vi "Set TCP Info.vi"(8 "error in (no error)":errorcluster, 10 "TCP Messaging Info":T1, 11 "Node in":refnum<class "Node.lvclass">) -> (0 "error out":errorcluster, 3 "Node out":refnum<class "Node.lvclass">)   [LabVIEW 2020, in "VolatusConfig.lvlib" / "Node.lvclass"]
uses:
  Node.lvclass
  Node.lvclass/Node.ctl
  VolatusConfigElement/VolatusConfigElement.lvclass
  lv-cdm/CDM-Config/Config Element/Config Element.lvclass
  lv-cdm/CDM-Config/Value Type.ctl
  lv-cdm/CDM-Config/CDM-Config.lvlib
  C:/dev/lv20CE/relink/lv-volatus/VolatusConfig/VolatusConfigElement/VolatusConfigElement.lvclass
  C:/dev/lv20CE/relink/lv-volatus/VolatusConfig/Node/Node.lvclass
  lv-vecto/Vecto/Node Config/TCP Messaging Info.ctl
  lv-vecto/VectoConfig/VectoConfig.lvlib
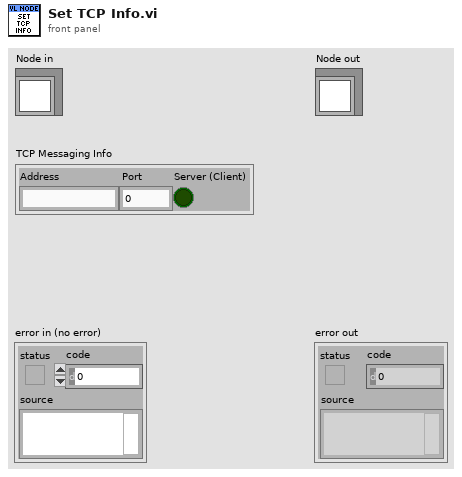
[diagram p1: front panel]
types:
  T1 = typedef "VectoConfig.lvlib/TCP Messaging Info.ctl" = cluster{"Address":string, "Port":u16, "Server (Client)":bool}
  T2 = typedef "CDM-Config.lvlib/Value Type.ctl" = enum16{"String", "Number", "Bool", "Object", "Array"}
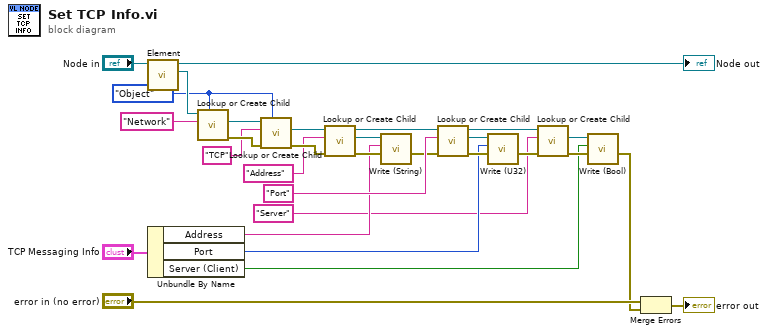
[diagram p0: block diagram]
diagram:
  w23 = Value_Type."Object" ("Value Type (String)")
  n1 = call "Element.vi"("VolatusConfigElement in"="Node in") -> ("Element"=w26:refnum<class "Config Element.lvclass">, "VolatusConfigElement out"=→"Node out":refnum<class "Node.lvclass">)  [unwired: 9 in]
  n2 = Unbundle By Name("TCP Messaging Info") -> ("Address"=w13:string, "Port"=w10:u16, "Server (Client)"=w5:bool)
  n3 = call "Lookup or Create Child.vi"("Value Type (Object)"=w23, "Name"="Network", "Config Element in"=w26) -> ("error out"=w29:errorcluster, "Child"=w24:refnum<class "Config Element.lvclass">)  [unwired: 5 in, 2 out]
  n4 = call "Lookup or Create Child.vi"("Value Type (Object)"=w23, "error in (no error)"=w29, "Name"="TCP", "Config Element in"=w24) -> ("error out"=w20:errorcluster, "Child"=w21:refnum<class "Config Element.lvclass">)  [unwired: 4 in, 2 out]
  n5 = call "Lookup or Create Child.vi"("error in (no error)"=w20, "Name"="Address", "Config Element in"=w21) -> ("error out"=w30:errorcluster, "Child"=w15:refnum<class "Config Element.lvclass">, "Config Element out"=w19:refnum<class "Config Element.lvclass">)  [unwired: 5 in, 1 out]
  n6 = call "Write (String).vi"("error in (no error)"=w30, "String Value"=w13, "Config Element in"=w15) -> ("error out"=w16:errorcluster)  [unwired: 7 in, 1 out]
  n7 = call "Lookup or Create Child.vi"("error in (no error)"=w16, "Name"="Port", "Config Element in"=w19) -> ("error out"=w12:errorcluster, "Child"=w11:refnum<class "Config Element.lvclass">, "Config Element out"=w8:refnum<class "Config Element.lvclass">)  [unwired: 5 in, 1 out]
  n8 = call "Write (U32).vi"("error in (no error)"=w12, "U32 Value"=w10, "Config Element in"=w11) -> ("error out"=w9:errorcluster)  [unwired: 7 in, 1 out]
  n9 = call "Lookup or Create Child.vi"("error in (no error)"=w9, "Name"="Server", "Config Element in"=w8) -> ("error out"=w7:errorcluster, "Child"=w6:refnum<class "Config Element.lvclass">)  [unwired: 5 in, 2 out]
  n10 = call "Write (Bool).vi"("error in (no error)"=w7, "Bool Value"=w5, "Config Element in"=w6) -> ("error out"=w2:errorcluster)  [unwired: 7 in, 1 out]
  n11 = Merge Errors("error in (no error)", w2) -> (→"error out":errorcluster)
